vi "Set Enable Averaging.vi"(8 "error in (no error)":errorcluster, 10 "Enable Averaging":bool, 11 "niDTS GNSS Dut in":refnum<class "niDTS GNSS Dut.lvclass">) -> (0 "error out":errorcluster, 3 "niDTS GNSS Dut out":refnum<class "niDTS GNSS Dut.lvclass">)   [LabVIEW 2015, in "niDTS GNSS.lvlib" / "niDTS GNSS Dut.lvclass"]
uses:
  niDTS GNSS Dut.lvclass
  niDTS GNSS Dut.lvclass/niDTS GNSS Dut.ctl
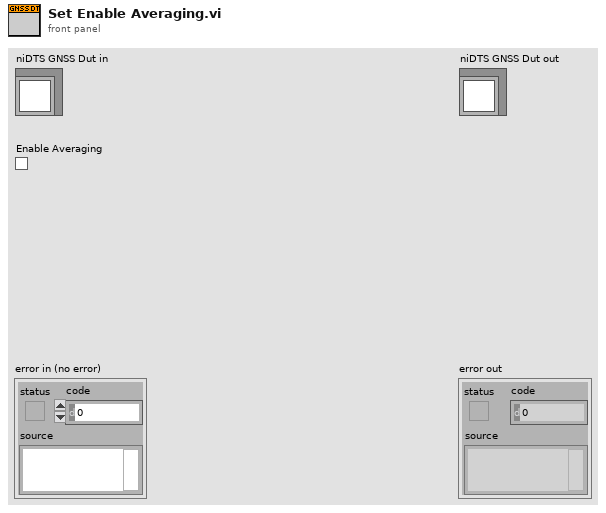
[diagram p1: front panel]
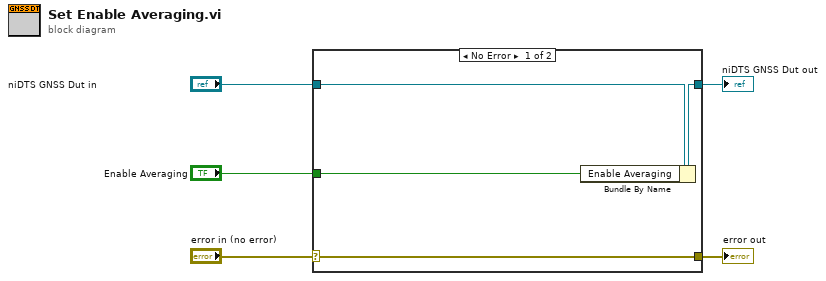
[diagram p0: block diagram]
diagram:
  n1 = case shown="No Error" "error in (no error)" {
    selector: "error in (no error)" -> [w9 w10]
    tunnel: [w9 w10] -> w4
    tunnel: [w7 w11] -> w2
    tunnel: "niDTS GNSS Dut in" -> [w8 w11]
    tunnel: "Enable Averaging" -> [w6 _]
    frame No Error {
      n2 = Bundle By Name(cluster=w8, "Enable Averaging"=w6) -> (w7:refnum<class "niDTS GNSS Dut.lvclass">)
    }
    frame Error {
    }
  }
  "error out" <- w4
  "niDTS GNSS Dut out" <- w2
